vi "get_pick_line_node_term.vi"(0 "Terms[] In":refnum<vi>[](array[refnum]), 11 "error in (no error)":errorcluster) -> (4 "Terms[]  Out":refnum<vi>[](array[refnum]), 6 "Pick Term":refnum<vi>, 8 "Multiline Term":refnum<vi>, 10 "Output Ref":refnum<vi>, 15 "error out":errorcluster)   [LabVIEW 2018]
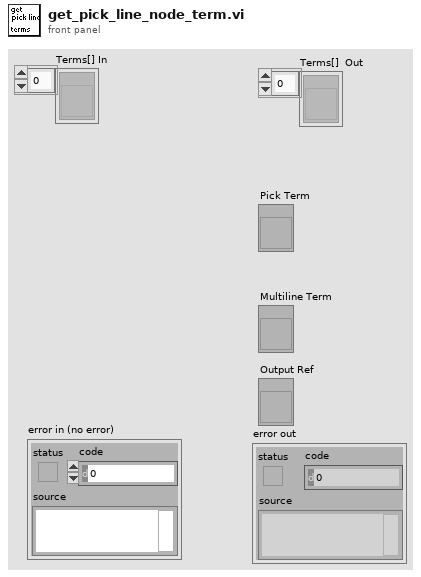
[diagram p1: front panel]
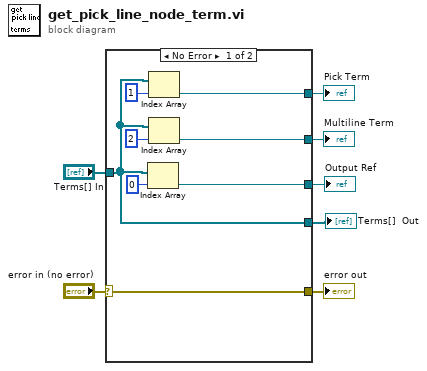
[diagram p0: block diagram]
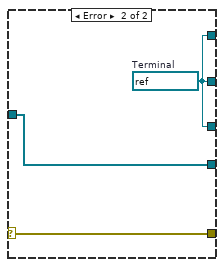
[diagram p2: hidden frame]
diagram:
  n1 = case shown="No Error" "error in (no error)" {
    selector: "error in (no error)" -> [w11 w18]
    tunnel: [w12 w16] -> w7
    tunnel: "Terms[] In" -> [w10 w17]
    tunnel: [w13 w16] -> w5
    tunnel: [w11 w18] -> w3
    tunnel: [w10 w17] -> w2
    tunnel: [w8 w16] -> w1
    frame No Error {
      n2 = Index Array(array=w10, index=0) -> (element=w8:refnum<vi>)
      n3 = Index Array(array=w10, index=1) -> (element=w12:refnum<vi>)
      n4 = Index Array(array=w10, index=2) -> (element=w13:refnum<vi>)
    }
    frame Error {
      w16 = refnum<vi> refnum  # Terminal
    }
  }
  "Pick Term" <- w7
  "Multiline Term" <- w5
  "error out" <- w3
  "Terms[]  Out" <- w2
  "Output Ref" <- w1
